vi "XOR Encryption - (1) Sender and Receiver Shared Key.vi"() -> ()   [LabVIEW 2013]
panel:
  out "Data Out":string
  in  "Data In":string
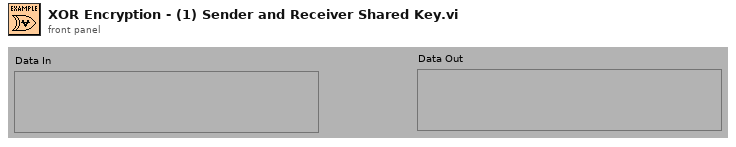
[diagram p1: front panel]
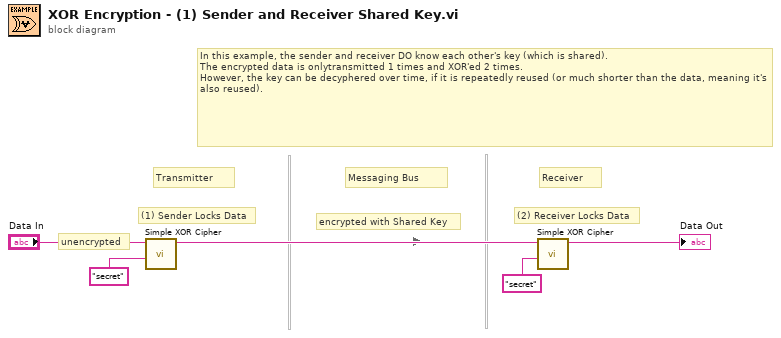
[diagram p0: block diagram]
diagram:
  # "Messaging Bus"
  # "Receiver"
  # "Transmitter"
  # "unencrypted"
  # "In this example, the sender and receiver DO know each other's key (which is shared).\nThe encrypted data is onlytransmitted 1 times and XOR'ed 2 times.\nHowever, the key can be decyphered over time, if it is repeatedly reused (or much shorter than the data, meaning it's also reused)."
  # "encrypted with Shared Key"
  # "(2) Receiver Locks Data"
  # "(1) Sender Locks Data"
  n1 = call "Simple XOR Cipher.vi"("key (\"\": random)"="secret", "data in"="Data In") -> ("data out"=w3:string)  [unwired: 8 in, 1 out]
  n2 = call "Simple XOR Cipher.vi"("key (\"\": random)"="secret", "data in"=w3) -> ("data out"=→"Data Out":string)  [unwired: 8 in, 1 out]
